vi "S7 TCP Test3.vi"() -> ()   [LabVIEW 2017]
uses:
  S7 TCP API Library/S7 Read Write Cluster.ctl
  S7 TCP API Library/Data Type.ctl
  S7 TCP API Library/S7 TCP.lvlib
panel:
  in  "Logging Config File Location":path=path "c:/config.csv"
  out "IP Address":string="172.16.102.180"
  out "Loop Time":dbl
  in  "milliseconds to wait":u32=100
  out "Data Valid Array":bool[](array[boolean])
  out "Output Data":dbl[](array[numeric])
  out "S7 Read Write Array":T1[](array[typedef])=[{"Read / Write"=4, "Address Areas"=132, "Data Block #"=0, "Start Address (bytes)"=10, "Data Type"=enum."Word (U16)", "Bit Number / Byte Length"=0, "Write Data"=0.0}, {"Read / Write"=4, "Address Areas"=132, "Data Block #"=0, "Start Address (bytes)"=201, "Data Type"=enum."Bit", "Bit Number / Byte Length"=7, "Write Data"=0.0}, {"Read / Write"=4, "Address Areas"=132, "Data Block #"=0, "Start Address (bytes)"=201, "Data Type"=enum."Byte (U8)", "Bit Number / Byte Length"=0, "Write Data"=0.0}, {"Read / Write"=4, "Address Areas"=132, "Data Block #"=0, "Start Address (bytes)"=201, "Data Type"=enum."Real (SGL)", "Bit Number / Byte Length"=0, "Write Data"=0.0}, {"Read / Write"=4, "Address Areas"=132, "Data Block #"=1, "Start Address (bytes)"=201, "Data Type"=enum."Byte (U8)", "Bit Number / Byte Length"=0, "Write Data"=0.0}, {"Read / Write"=4, "Address Areas"=132, "Data Block #"=1, "Start Address (bytes)"=201, "Data Type"=enum."Signed Byte (I8)", "Bit Number / Byte Length"=0, "Write Data"=0.0}] {"Address Areas" items=["I/O (P)"=128, "Input (I)"=129, "Output (Q)"=130, "Bit Memory (M)"=131, "Data (DB)"=132, "Instance Data (DI)"=133, "Local Data (L)"=134, "Predecessor Local Data (VL)"=135]; "Read / Write" items=["Read"=4, "Write"=5]; "Bit Number / Byte Length" max=7 step=1}
  out "Loop Itteration":i32
  in  "Stop":bool
  out "error out":errorcluster
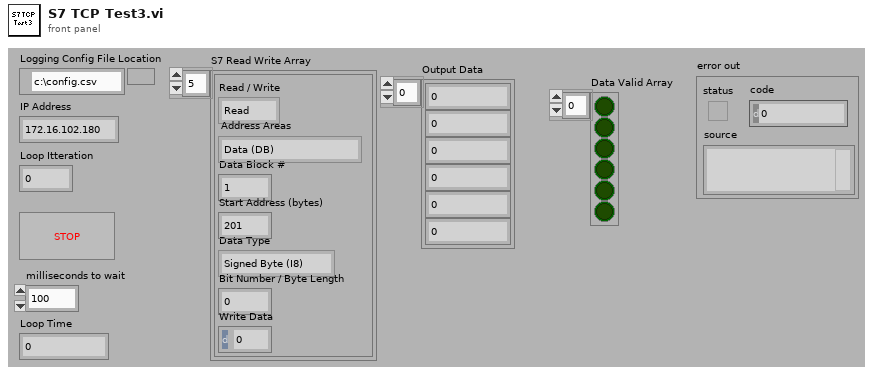
[diagram p1: front panel]
types:
  T1 = typedef "S7 TCP.lvlib/S7 Read Write Cluster.ctl" = cluster{"Read / Write":u8, "Address Areas":u8, "Data Block #":u16, "Start Address (bytes)":u32, "Data Type":T2, "Bit Number / Byte Length":u8, "Write Data":dbl}
  T2 = typedef "S7 TCP.lvlib/Data Type.ctl" = enum16{"Bit", "Byte (U8)", "Signed Byte (I8)", "Word (U16)", "Signed Word (I16)", "Long (U32)", "Signed Long (I32)", "Real (SGL)", "Defined Byte Length"}
  T3 = typedef "S7 TCP.lvlib/Optimized Data Index.ctl" = cluster{"DB Index":i32, "Data Index":i32, "Length":i32, "Data Type":T2, "Bit Number":u8}
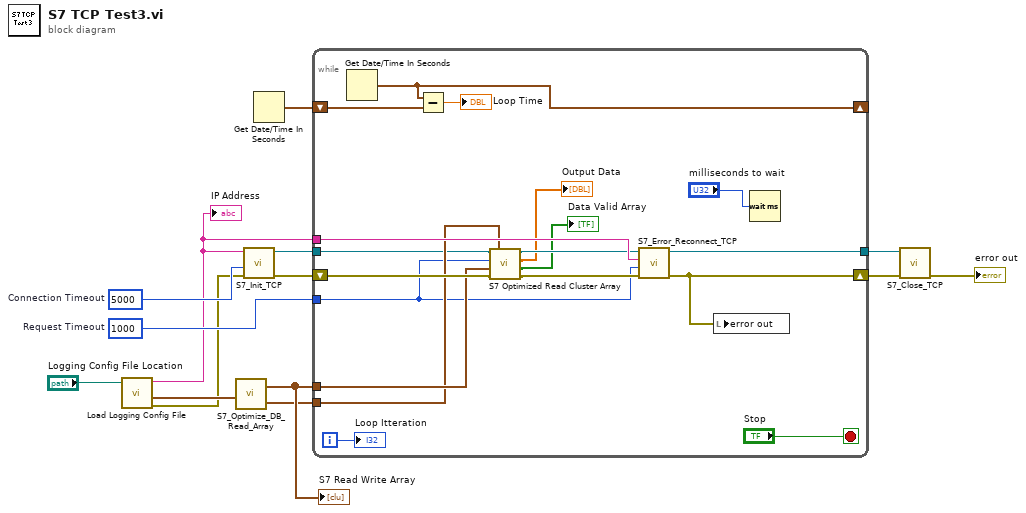
[diagram p0: block diagram]
diagram:
  w8 = u32 1000  # Request Timeout
  w12 = u32 5000  # Connection Timeout
  n1 = call "Load Logging Config File.vi"("Logging Config File Location"="Logging Config File Location") -> ("IP Address"=w3:string, "S7 Read Write Array"=w5:T1[], "error out"=w4:errorcluster)  [unwired: 1 in, 2 out]
  "IP Address" <- w3
  n2 = call "S7_Optimize_DB_Read_Array.vi"("S7 Read Array Input"=w5) -> ("Optimized Data Index"=w1:T3[], "Optimized S7 Read Array Output"=w2:T1[])  [unwired: 1 in]
  "S7 Read Write Array" <- w2
  n3 = call "S7_Init_TCP.vi"("error in"=w4, "Connection Timeout"=w12, "IP Address"=w3) -> ("error out"=w10:errorcluster, "TCP Connection Ref"=w9:refnum<k5>)  [unwired: 2 in, 5 out]
  n4 = Get Date/Time In Seconds() -> (seconds since 1Jan1904=w7:timestamp)
  n5 = while {
    tunnel: w9 -> [w18]
    tunnel: [w29] -> w14
    tunnel: w8 -> [w19]
    shift-right: [w30] -> w11
    shift-left: w10 -> [w23]
    shift-right: [w26] -> _
    shift-left: w7 -> [w27]
    tunnel: w2 -> [w21]
    tunnel: w3 -> [w24]
    tunnel: w1 -> [w20]
    i -> [w31]
    stop <- "Stop" stop-if-true
    n6 = Get Date/Time In Seconds() -> (seconds since 1Jan1904=w26:timestamp)
    n7 = Subtract(x=w26, y=w27) -> (x-y=→"Loop Time":dbl)
    n8 = call "S7 Optimized Read Cluster Array.vi"("Optimized Data Index"=w20, "error in"=w23, "S7 Optimized Read Array"=w21, "Timeout"=w19, "TCP Connection Ref"=w18) -> ("error out"=w22:errorcluster, "Data Valid Array"=→"Data Valid Array":bool[], "Output Data"=→"Output Data":dbl[], "TCP Connection Ref Out"=w17:refnum<k5>)  [unwired: 3 out]
    n9 = call "S7_Error_Reconnect_TCP.vi"("error in"=w22, "Timeout"=w19, "IP Address"=w24, "TCP Connection Ref"=w17) -> ("error out"=w30:errorcluster, "TCP Connection Ref Out"=w29:refnum<k5>)  [unwired: 6 out]
    n10 = local write "error out"(w30) -> ()
    n11 = Wait (ms)(milliseconds to wait="milliseconds to wait") -> ()  [unwired: 1 out]
    "Loop Itteration" <- w31
  }
  n12 = call "S7_Close_TCP.vi"("error in"=w11, "TCP Connection Ref"=w14) -> ("error out"=→"error out":errorcluster)  [unwired: 1 in, 8 out]
